vi "Module.Window, Set Pane Size.vi"(9 "Height-Width":cluster{"W":i16, "H":i16}, 10 "VI Ref VI":refnum<vi>, 11 "Sys":T1) -> (0 "error out":errorcluster)   [LabVIEW 2024, in "EQMF.lvlib" / "Module Utils.lvlib"]
uses:
  Module Utils.lvlib
  Module Sys Info.ctl
  Config/Stored Controls/Class.SaveCtrls.lvclass
  Event Log/Event Notification/Event Notification.lvclass
  Config/App Data/Class.AppData.lvclass
  Subscription/Subscription.lvclass
  Queues/Q.Element.ctl
  Module.SW Version Info.ctl
  Module Config.ctl
  Module.Working Dirs.ctl
  Queues/Queue Utils.lvlib
panel:
  # "Name, PN, Version, Note"
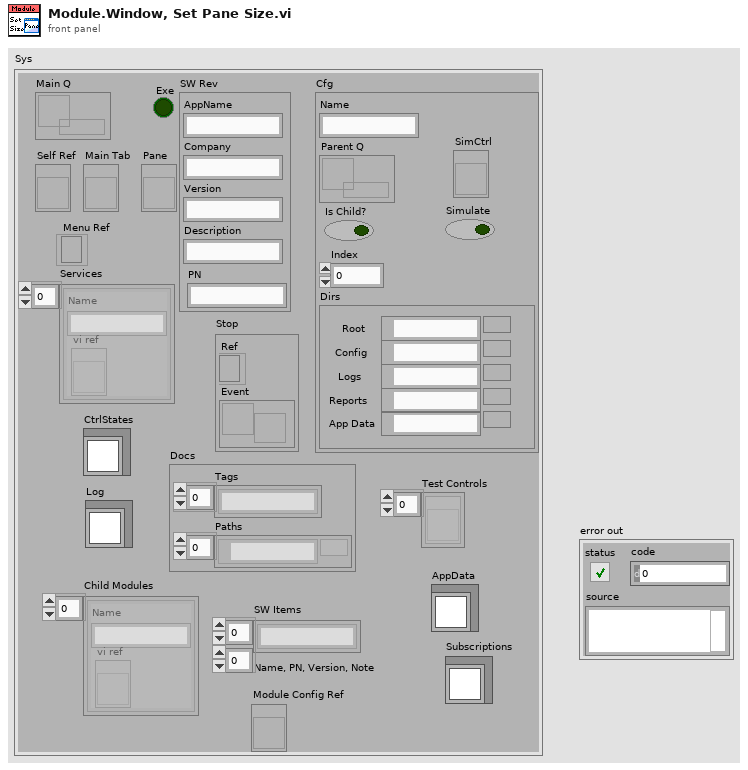
[diagram p1: front panel]
types:
  T1 = typedef "EQMF.lvlib/Module Utils.lvlib/Module Sys Info.ctl" = cluster{"Main Q":refnum<queue>, "Exe":bool, "SW Rev":T2, "Self Ref":refnum<vi>, "Main Tab":refnum<vi>, "Pane":refnum<vi>, "Stop":cluster{"Ref":refnum<event-registration>, "Event":refnum<user-event>}, "Cfg":T3, "Services":cluster{"Name":string, "vi ref":refnum<vi>}[], "Menu Ref":refnum<k9>, "CtrlStates":refnum<class "Class.SaveCtrls.lvclass">, "Docs":cluster{"Tags":string[], "Paths":path[]}, "Log":refnum<class "Event Notification.lvclass">, "Test Controls":refnum<vi>[], "Child Modules":cluster{"Name":string, "vi ref":refnum<vi>}[], "SW Items":string[][], "AppData":refnum<class "Class.AppData.lvclass">, "Subscriptions":refnum<class "Subscription.lvclass">, "Module Config Ref":refnum<vi>}
  T2 = typedef "EQMF.lvlib/Module Utils.lvlib/Module.SW Version Info.ctl" = cluster{"AppName":string, "Company":string, "Version":string, "Description":string, "PN":string}
  T3 = typedef "EQMF.lvlib/Module Utils.lvlib/Module Config.ctl" = cluster{"Name":string, "Parent Q":refnum<queue>, "Is Child?":bool, "Index":i32, "Dirs":T4, "Simulate":bool, "SimCtrl":refnum<vi>}
  T4 = typedef "EQMF.lvlib/Module Utils.lvlib/Module.Working Dirs.ctl" = cluster{"Root":path, "Config":path, "Logs":path, "Reports":path, "App Data":path}
  T5 = typedef "EQMF.lvlib/Queue Utils.lvlib/Q.Element.ctl" = cluster{"Cmd":string, "Sub":string, "Data1":variant, "Data2":variant}
  T6 = typedef "LVRectTypeDef.ctl" = cluster{"Left":i16, "Top":i16, "Right":i16, "Bottom":i16}
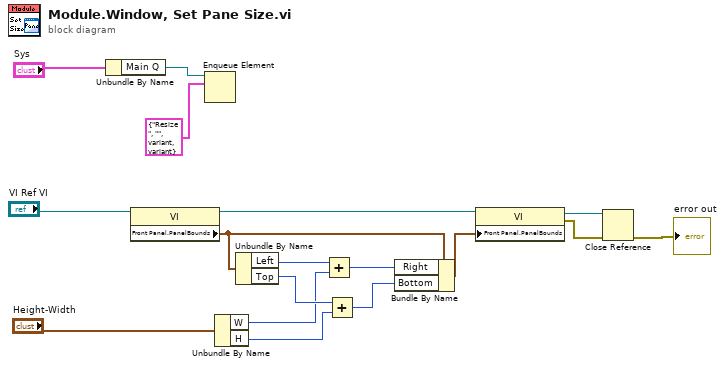
[diagram p0: block diagram]
diagram:
  n1 = Unbundle By Name("Sys") -> ("Main Q"=w5:refnum<queue>)
  n2 = property class="VI"(reference="VI Ref VI") -> (reference out=w10:refnum<vi>, "Front Panel.PanelBounds"=w9:T6)  [unwired: 1 in, 1 out]
  n3 = Enqueue Element(queue=w5, element=T5 {"Cmd"="Resize", "Sub"="", "Data1"=variant, "Data2"=variant}) -> ()  [unwired: 2 in, 3 out]
  n4 = Unbundle By Name("Height-Width") -> ("W"=w12:i16, "H"=w11:i16)
  n5 = Unbundle By Name(w9) -> ("Left"=w16:i16, "Top"=w15:i16)
  n6 = Add(x=w16, y=w12) -> (x+y=w14:i16)
  n7 = Add(x=w15, y=w11) -> (x+y=w13:i16)
  n8 = Bundle By Name(cluster=w9, "Right"=w14, "Bottom"=w13) -> (w17:T6)
  n9 = property class="VI"(reference=w10, "Front Panel.PanelBounds"=w17) -> (reference out=w8:refnum<vi>, error out=w7:errorcluster)  [unwired: 1 in]
  n10 = Close Reference(reference=w8, error in (no error)=w7) -> (error out=→"error out":errorcluster)
